vi "GetHSSpeedSD.vi"(4 "error in (no error)":errorcluster, 5 "index":i32, 6 "type":T1, 7 "channel":i32) -> (0 "error out":errorcluster, 1 "DLL error code":u32, 2 "speed":sgl format="%.2f")   [LabVIEW 2015]
doc: "As your AndorMCD[tm] system is capable of operating at more than one horizontal shift speed this function will return the actual speeds available. The value returned is in microseconds per pixel shift.\n\n<B>Parameters:</B>\nchannel - the AD channel\ntype - the horizontal read mode\n Valid values: 0 - speed of data readout\n 1 - speed of binning\n 2 - speed of dumping pixels\nindex - speed required\n Valid values: 0 to <B>GetNumberHSSpeeds</B>-1\nspeed - speed in micro-seconds per pixel shift\n\n<B>Error codes:</B>\nDRV_SUCCESS - Speed returned.\nDRV_NOT_INITIALIZED - System not initialized.\nDRV_ACQUIRING - Acquisition in progress.\nDRV_P1INVALID - Invalid channel.\nDRV_P2INVALID - Invalid horizontal read mode.\nDRV_P3INVALID - Invalid index."
uses:
  atmcd32d.llb/HSSpeed_type typedef.ctl
  DLL/atmcd32d.dll
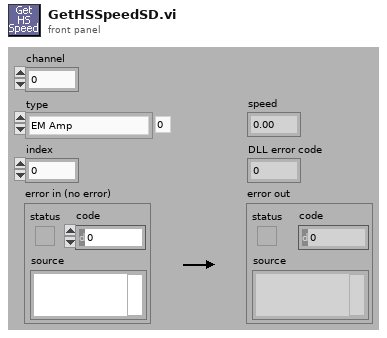
[diagram p1: front panel]
types:
  T1 = typedef "HSSpeed_type typedef.ctl" = enum16{"EM Amp", "Conventional Amp"}
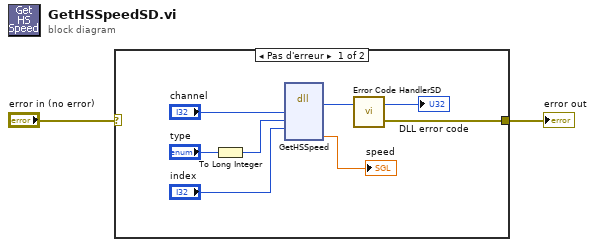
[diagram p0: block diagram]
diagram:
  n1 = case shown="Pas d'erreur" "error in (no error)" {
    selector: "error in (no error)" -> [_ w11]
    tunnel: [w9 w11] -> w1
    frame No Error {
      n2 = To Long Integer(number="type") -> (32bit integer=w5:i32)
      n3 = dll-call lib="G:/SD/TRANCON-2015/DLL/Atmcd32d.dll" fn="GetHSSpeed"("channel"="channel", "type"=w5, "index"="index") -> (w10:u32, "speed"=→"speed":sgl)  [unwired: 7 in, 2 out]
      n4 = call "Error Code HandlerSD.vi"("DLL error code"=w10) -> ("error out"=w9:errorcluster, "dup DLL error code"=→"DLL error code":u32)  [unwired: 1 in]
    }
    frame Error {
    }
  }
  "error out" <- w1
